vi "Lockin Global.vi"() -> ()   [LabVIEW 2009, in "Lockin.lvclass"]
uses:
  Lockin.lvclass
panel:
  out "timeconst":cluster{"tcstring":string, "tcnum":dbl}[](array[cluster])=[{"tcstring"="10 microsec", "tcnum"=1e-05}, {"tcstring"="30 microsec", "tcnum"=3e-05}, {"tcstring"="100 microsec", "tcnum"=0.0001}, {"tcstring"="300 microsec", "tcnum"=0.0003}, {"tcstring"="1 ms", "tcnum"=0.001}, {"tcstring"="3 ms", "tcnum"=0.003}, {"tcstring"="10 ms", "tcnum"=0.01}, {"tcstring"="30 ms", "tcnum"=0.03}, {"tcstring"="100 ms", "tcnum"=0.1}, {"tcstring"="300 ms", "tcnum"=0.3}, {"tcstring"="1 s", "tcnum"=1.0}, {"tcstring"="3 s", "tcnum"=3.0}, {"tcstring"="10 s", "tcnum"=10.0}, {"tcstring"="30 s", "tcnum"=30.0}, {"tcstring"="100 s", "tcnum"=100.0}, {"tcstring"="300 s", "tcnum"=300.0}, {"tcstring"="1 ks", "tcnum"=1000.0}, {"tcstring"="3 ks", "tcnum"=3000.0}, {"tcstring"="10 ks", "tcnum"=10000.0}, {"tcstring"="30 ks", "tcnum"=30000.0}]
  out "sens":cluster{"sensstring":string, "sensenum":dbl}[](array[cluster])=[{"sensstring"="2 nV", "sensenum"=2e-09}, {"sensstring"="5 nV", "sensenum"=5e-09}, {"sensstring"="10 nV", "sensenum"=1e-08}, {"sensstring"="20 nV", "sensenum"=2e-08}, {"sensstring"="50 nV", "sensenum"=5e-08}, {"sensstring"="100 nV", "sensenum"=1e-07}, {"sensstring"="200 nV", "sensenum"=2e-07}, {"sensstring"="500 nV", "sensenum"=5e-07}, {"sensstring"="1 microV", "sensenum"=1e-06}, {"sensstring"="2 microV", "sensenum"=2e-06}, {"sensstring"="5 microV", "sensenum"=5e-06}, {"sensstring"="10 microV", "sensenum"=1e-05}, {"sensstring"="20 microV", "sensenum"=2e-05}, {"sensstring"="50 microV", "sensenum"=5e-05}, {"sensstring"="100 microV", "sensenum"=0.0001}, {"sensstring"="200 microV", "sensenum"=0.0002}, {"sensstring"="500 microV", "sensenum"=0.0005}, {"sensstring"="1 mV", "sensenum"=0.001}, {"sensstring"="2 mV", "sensenum"=0.002}, {"sensstring"="5 mV", "sensenum"=0.005}, {"sensstring"="10 mV", "sensenum"=0.01}, {"sensstring"="20 mV", "sensenum"=0.02}, {"sensstring"="50 mV", "sensenum"=0.05}, {"sensstring"="100 mV", "sensenum"=0.1}, {"sensstring"="200 mV", "sensenum"=0.2}, {"sensstring"="500 mV", "sensenum"=0.5}, {"sensstring"="1 V", "sensenum"=1.0}]
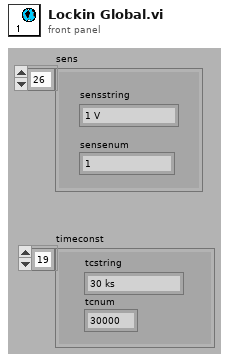
[diagram p1: front panel]
diagram:
